vi "CAN_setOutput.vi"(8 "error in (no error)":errorcluster, 9 "Output Right":dbl, 10 "Output Left":dbl, 11 "CAN Jaguars Ref":T1) -> (0 "error out":errorcluster, 3 "CAN Jaguars Ref out":T1)   [LabVIEW 2009, in "OWNCAN.lvlib"]
doc: "Sets output of left and right Jaguar controllers."
uses:
  OWNCAN.lvlib
  CAN Jaguars Ref.ctl
  CAN/SubVIs/CAN Jaguar Ref.ctl
  CAN/SubVIs/CAN Jaguar Control Mode.ctl
  CAN.lvlib
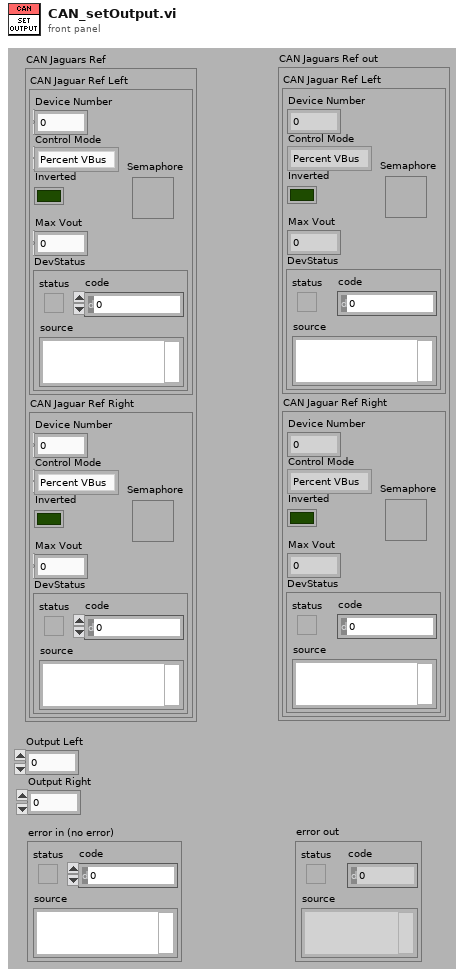
[diagram p1: front panel]
types:
  T1 = typedef "OWNCAN.lvlib/CAN Jaguars Ref.ctl" = cluster{"CAN Jaguar Ref Left":T2, "CAN Jaguar Ref Right":T2}
  T2 = typedef "CAN.lvlib/CAN Jaguar Ref.ctl" = cluster{"Device Number":u8, "Control Mode":T3, "Inverted":bool, "Semaphore":T4, "Max Vout":dbl, "DevStatus":errorcluster}
  T3 = typedef "CAN.lvlib/CAN Jaguar Control Mode.ctl" = enum16{"Percent VBus", "Speed", "Position", "Current"}
  T4 = typedef "Semaphore RefNum" = refnum<k1>
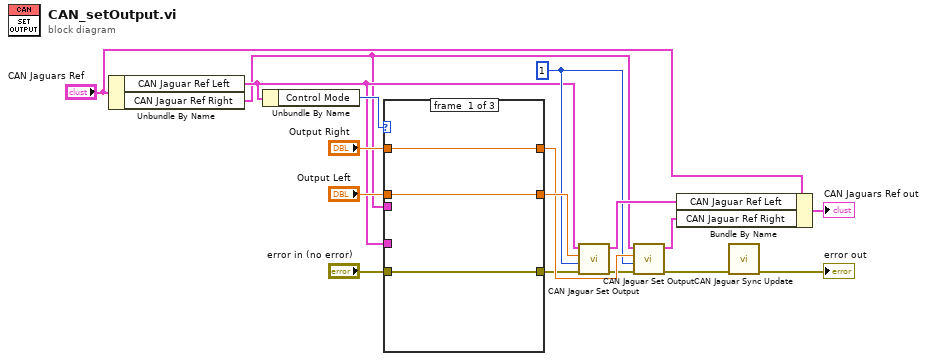
[diagram p0: block diagram]
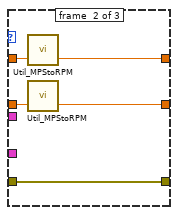
[diagram p2: hidden frame]
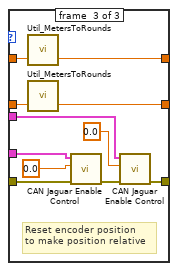
[diagram p3: hidden frame]
diagram:
  w8 = u8 1 ("Sync group bit mask")
  n1 = Unbundle By Name("CAN Jaguars Ref") -> ("CAN Jaguar Ref Left"=w6:T2, "CAN Jaguar Ref Right"=w5:T2)
  n2 = Unbundle By Name(w6) -> ("Control Mode"=w17:T3)
  n3 = case shown="\"Percent VBus\", Default" w17 {
    tunnel: "Output Left" -> [w19 w25 w36]
    tunnel: [w19 w24 w35] -> w15
    tunnel: "Output Right" -> [w20 w23 w34]
    tunnel: [w20 w22 w33] -> w13
    tunnel: w6 -> [_ _ w32]
    tunnel: w5 -> [_ _ w30]
    tunnel: "error in (no error)" -> [w18 w21 w28]
    tunnel: [w18 w21 w26] -> w3
    frame #0 {
    }
    frame #1 {
      n4 = call "Util_MPStoRPM.vi"("m/s robot"=w23) -> ("rpm gear"=w22:dbl)  [unwired: 2 in]
      n5 = call "Util_MPStoRPM.vi"("m/s robot"=w25) -> ("rpm gear"=w24:dbl)  [unwired: 2 in]
    }
    frame #2 {
      # "Reset encoder position\nto make position relative"
      n6 = call "Util_MetersToRounds.vi"("distance (m) robot"=w34) -> ("rotations gear"=w33:dbl)  [unwired: 2 in]
      n7 = call "Util_MetersToRounds.vi"("distance (m) robot"=w36) -> ("rotations gear"=w35:dbl)  [unwired: 2 in]
      n8 = call "CAN Jaguar Enable Control.vi"("error in (no error)"=w28, "Encoder Initial Position"=0.0, "CAN Jaguar Ref"=w32) -> ("error out"=w27:errorcluster)  [unwired: 7 in, 1 out]
      n9 = call "CAN Jaguar Enable Control.vi"("error in (no error)"=w27, "Encoder Initial Position"=0.0, "CAN Jaguar Ref"=w30) -> ("error out"=w26:errorcluster)  [unwired: 7 in, 1 out]
    }
  }
  n10 = call "CAN Jaguar Set Output.vi"("error in (no error)"=w3, "Sync group bit mask"=w8, "Output Set Point"=w15, "CAN Jaguar Ref"=w6) -> ("error out"=w2:errorcluster, "CAN Jaguar Ref Out"=w11:T2)  [unwired: 6 in]
  n11 = call "CAN Jaguar Set Output.vi"("error in (no error)"=w2, "Sync group bit mask"=w8, "Output Set Point"=w13, "CAN Jaguar Ref"=w5) -> ("error out"=w1:errorcluster, "CAN Jaguar Ref Out"=w12:T2)  [unwired: 6 in]
  n12 = Bundle By Name(cluster="CAN Jaguars Ref", "CAN Jaguar Ref Left"=w11, "CAN Jaguar Ref Right"=w12) -> (→"CAN Jaguars Ref out":T1)
  n13 = call "CAN Jaguar Sync Update.vi"("error in (no error)"=w1) -> ("error out"=→"error out":errorcluster)  [unwired: 10 in]
